vi "LED.vi"(2 "error in (no error)":errorcluster, 3 "Enum":T1(ring)=enum."Initialize") -> (0 "error out":errorcluster)   [LabVIEW 2017]
uses:
  <vilib>/myRIO/Instrument Drivers/Onboard IO/DIO/typedefs/DIO Reference.ctl
  <vilib>/myRIO/Common/Instrument Driver Framework/Utilities/typedefs/myRIO Generic Hardware Reference.ctl
  <vilib>/myRIO/Common/Instrument Driver Framework/Utilities/typedefs/Hardware Version Enum.ctl
  <vilib>/myRIO/Common/Instrument Driver Framework/Utilities/typedefs/myRIO v1.0 Reference.ctl
  <vilib>/myRIO/Common/Instrument Driver Framework/Utilities/typedefs/Generic FPGA Reference.ctl
  <vilib>/myRIO/Common/Instrument Driver Framework/myRIO v1.0/DIO/typedefs/DIO Channels List.ctl
  <vilib>/myRIO/Common/Instrument Driver Framework/myRIO v1.0/DIO/typedefs/DIO Channels Enum.ctl
  <vilib>/userdefined/High Color/nirio_resource_hc.ctl
  <vilib>/myRIO/Common/Instrument Driver Framework/Utilities/vis/Is FPGA Ref Available.vi
  <vilib>/myRIO/Common/Instrument Driver Framework/myRIO v1.0/DIO/vis/myRIO v1.1 Open DIO.vi
  <vilib>/myRIO/Instrument Drivers/Onboard IO/DIO/vis/Write.vi
  <vilib>/myRIO/Common/Instrument Driver Framework/Utilities/vis/Validate Channels.vi
  <vilib>/myRIO/Common/Instrument Driver Framework/myRIO v1.0/DIO/vis/myRIO v1.0 Reserve DIO.vi
  <vilib>/myRIO/Common/Instrument Driver Framework/myRIO v1.0/Resource Manager/vis/myRIO v1.0 Reserve Channel List.vi
  <vilib>/myRIO/Common/Instrument Driver Framework/myRIO v1.0/DIO/vis/myRIO v1.0 Build MUX Configuration DIO.vi
  <vilib>/myRIO/Common/Instrument Driver Framework/myRIO v1.0/Resource Manager/vis/myRIO v1.0 Reserve Channel.vi
  <vilib>/myRIO/Common/Instrument Driver Framework/myRIO v1.0/Resource Manager/vis/myRIO v1.0 Unreserve Channel.vi
  <vilib>/myRIO/Common/Instrument Driver Framework/myRIO v1.0/Resource Manager/vis/myRIO v1.0 Create Configuration List.vi
  <vilib>/myRIO/Common/Instrument Driver Framework/myRIO v1.0/Resource Manager/vis/myRIO v1.0 Build Mutex Name.vi
  <vilib>/Utility/VariantDataType/GetNumericInfo.vi
  <vilib>/Utility/error.llb/Error Cluster From Error Code.vi
  <vilib>/myRIO/Common/Instrument Driver Framework/myRIO v1.0/myRIO v1.1 Open.vi
  <vilib>/myRIO/Common/Instrument Driver Framework/Utilities/vis/IO Manager.vi
  <vilib>/myRIO/Common/Instrument Driver Framework/Utilities/vis/Configuration Manager.vi
  <vilib>/myRIO/Common/Instrument Driver Framework/myRIO v1.0/Resource Manager/vis/myRIO v1.0 Configure IO.vi
  <vilib>/myRIO/Common/Instrument Driver Framework/myRIO v1.0/myRIO v1.0 Close.vi
  <vilib>/myRIO/Common/Instrument Driver Framework/myRIO v1.0/DIO/vis/myRIO v1.0 Write DIO.vi
  <vilib>/myRIO/Express VI/Onboard Devices/LED/LED Express VI.xnode
  <vilib>/myRIO/Instrument Drivers/Onboard IO/DIO/vis/myRIO DIO Open.xnode
  <vilib>/myRIO/Instrument Drivers/Onboard IO/DIO/DIO.lvlib
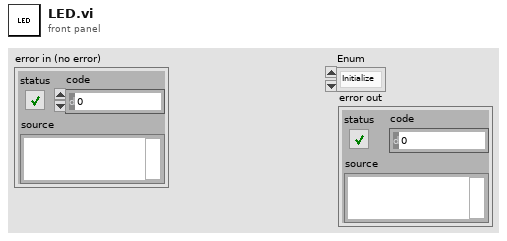
[diagram p1: front panel]
types:
  T1 = enum16{"Terminate", "Finalize", "Execute", "Initialize"}
  T2 = typedef "DIO.lvlib/DIO Reference.ctl" = cluster{"myRIO Reference":T3, "DIO Channels List":T7}
  T3 = typedef "myRIO Generic Hardware Reference.ctl" = cluster{"myRIO Model":T4, "myRIO Hardware Reference":T5}
  T4 = typedef "Hardware Version Enum.ctl" = enum16{"Unknown", "myRIO-1900", "myRIO-1950", "roboRIO", "NI ELVIS RIO CM"}
  T5 = typedef "myRIO v1.0 Reference.ctl" = cluster{"Generic FPGA Reference":T6, "Allow multiple opens":bool}
  T6 = typedef "Generic FPGA Reference.ctl" = refnum<k20>
  T7 = typedef "DIO Channels List.ctl" = T8[]
  T8 = typedef "DIO Channels Enum.ctl" = enum16{"Not Connected", "C/DIO0", "C/DIO1", "C/DIO2", "C/DIO3", "C/DIO4", "C/DIO5", "C/DIO6", "C/DIO7", "A/DIO0", "A/DIO1", "A/DIO2", "A/DIO3", "A/DIO4", "A/DIO5", "A/DIO6", "A/DIO7", "A/DIO8", "A/DIO9", "A/DIO10", "A/DIO11", "A/DIO12", "A/DIO13", "A/DIO14", "A/DIO15", "B/DIO0", "B/DIO1", "B/DIO2", "B/DIO3", "B/DIO4", "B/DIO5", "B/DIO6", "B/DIO7", "B/DIO8", "B/DIO9", "B/DIO10", "B/DIO11", "B/DIO12", "B/DIO13", "B/DIO14", "B/DIO15", "LED0", "LED1", "LED2", "LED3", "Button0", "DIO/DIO0", "DIO/DIO1", "DIO/DIO2", "DIO/DIO3", "DIO/DIO4", "DIO/DIO5", "DIO/DIO6", "DIO/DIO7", "DIO/DIO8", "DIO/DIO9", "SPI/CS0", "SPI/CS1", "SPI/CS2", "SPI/CS3", "LED RADIO (Green)", "LED RADIO (Red)", "LED COMM (Green)", "LED COMM (Red)", "LED MODE (Green)", "LED MODE (Red)"}
  T9 = typedef "nirio_resource_hc.ctl" = tag
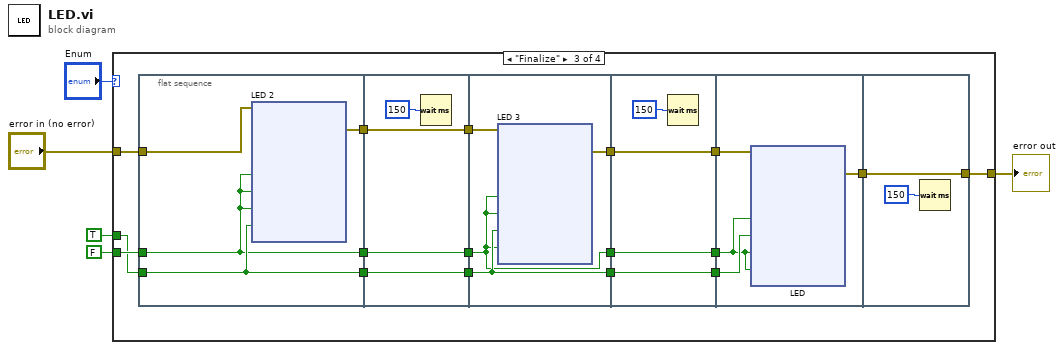
[diagram p0: block diagram]
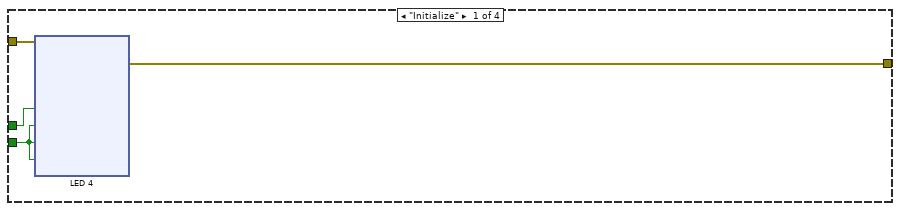
[diagram p2: hidden frame]
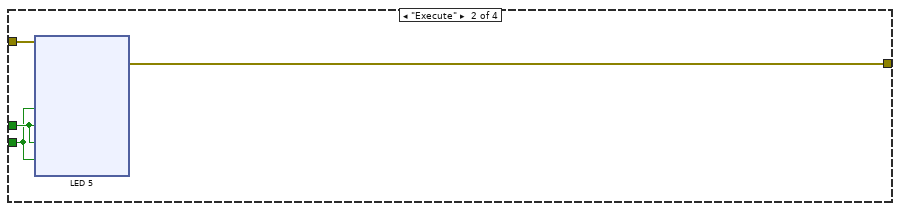
[diagram p3: hidden frame]
diagram:
  n1 = case shown="\"Finalize\"" "Enum" {
    tunnel: TRUE -> [w8 w51 w105 _]
    tunnel: FALSE -> [w9 w50 w106 _]
    tunnel: [w7 w49 w92 w243] -> w1
    tunnel: "error in (no error)" -> [w6 w48 w90 w243]
    frame "Initialize" {
      n2 = xnode "LED 4"("LED0"=w8, "LED1"=w9, "LED2"=w9, "LED3"=w9, "error in (no error)"=w6) -> ("error out"=w7:errorcluster)
    }
    frame "Execute" {
      n3 = xnode "LED 5"("LED0"=w50, "LED1"=w51, "LED2"=w51, "LED3"=w50, "error in (no error)"=w48) -> ("error out"=w49:errorcluster)
    }
    frame "Finalize" {
      n4 = flat-sequence {
        tunnel: w106 -> [w109]
        tunnel: w105 -> [w110]
        tunnel: [w110] -> w104
        tunnel: [w109] -> w102
        tunnel: [w108] -> w95
        tunnel: w90 -> [w107]
        tunnel: w104 -> [w152]
        tunnel: [w152] -> w103
        tunnel: w102 -> [w151]
        tunnel: [w151] -> w101
        tunnel: [w149] -> w96
        tunnel: w95 -> [w149]
        tunnel: w103 -> [w156]
        tunnel: w101 -> [w155]
        tunnel: [w156] -> w100
        tunnel: [w155] -> w98
        tunnel: w96 -> [w154]
        tunnel: [w153] -> w93
        tunnel: w100 -> [w198]
        tunnel: [w198] -> w99
        tunnel: w98 -> [w197]
        tunnel: [w197] -> w97
        tunnel: [w195] -> w94
        tunnel: w93 -> [w195]
        tunnel: w99 -> [w202]
        tunnel: w97 -> [w201]
        tunnel: w94 -> [w200]
        tunnel: [w199] -> w91
        tunnel: [w241] -> w92
        tunnel: w91 -> [w241]
        frame #0 {
          n5 = xnode "LED 2"("LED0"=w109, "LED1"=w109, "LED2"=w109, "LED3"=w110, "error in (no error)"=w107) -> ("error out"=w108:errorcluster)
        }
        frame #1 {
          n6 = Wait (ms)(milliseconds to wait=u32 150) -> ()  [unwired: 1 out]
        }
        frame #2 {
          n7 = xnode "LED 3"("LED0"=w155, "LED1"=w155, "LED2"=w156, "LED3"=w155, "error in (no error)"=w154) -> ("error out"=w153:errorcluster)
        }
        frame #3 {
          n8 = Wait (ms)(milliseconds to wait=u32 150) -> ()  [unwired: 1 out]
        }
        frame #4 {
          n9 = xnode "LED"("LED0"=w201, "LED1"=w202, "LED2"=w201, "LED3"=w201, "error in (no error)"=w200) -> ("error out"=w199:errorcluster)
        }
        frame #5 {
          n10 = Wait (ms)(milliseconds to wait=u32 150) -> ()  [unwired: 1 out]
        }
      }
    }
    frame "Terminate" {
    }
  }
  "error out" <- w1
